vi "Write bool.vi"(0 "OWEN HMI in":refnum<class "OWEN HMI.lvclass">, 5 "Bool":T1, 11 "error in (no error)":errorcluster) -> (4 "OWEN HMI out":refnum<class "OWEN HMI.lvclass">, 15 "error out":errorcluster)   [LabVIEW 2019, in "OWEN HMI.lvclass"]
uses:
  OWEN HMI.lvclass
  Bool data.ctl
  OWEN HMI.lvclass/OWEN HMI.ctl
  <vilib>/NI/Modbus Library/API/Master/Modbus Master.lvclass
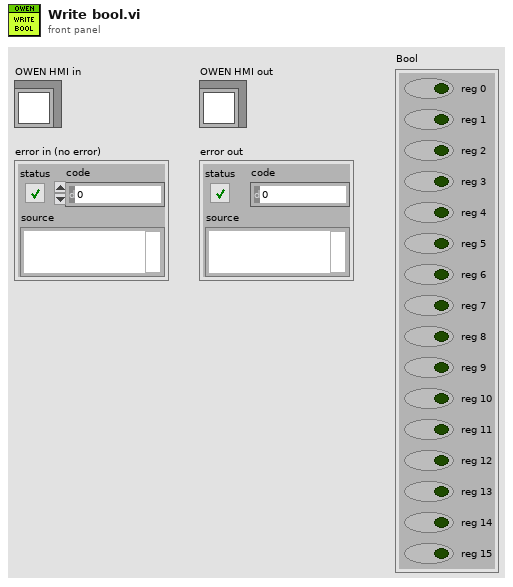
[diagram p1: front panel]
types:
  T1 = typedef "OWEN HMI.lvclass/Bool data.ctl" = cluster{"reg 0":bool, "reg 1":bool, "reg 2":bool, "reg 3":bool, "reg 4":bool, "reg 5":bool, "reg 6":bool, "reg 7":bool, "reg 8":bool, "reg 9":bool, "reg 10":bool, "reg 11":bool, "reg 12":bool, "reg 13":bool, "reg 14":bool, "reg 15":bool}
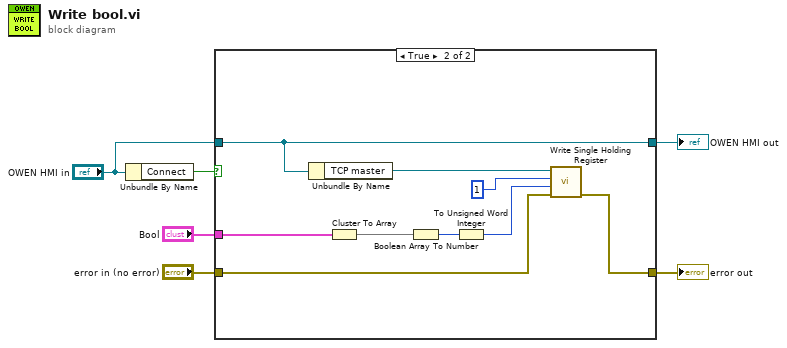
[diagram p0: block diagram]
diagram:
  n1 = Unbundle By Name("OWEN HMI in") -> ("Connect"=w6:bool)
  n2 = case shown="True" w6 {
    tunnel: "error in (no error)" -> [w8 w10]
    tunnel: "OWEN HMI in" -> [w7 w17]
    tunnel: [w7 w17] -> w3
    tunnel: [w8 w9] -> w2
    tunnel: "Bool" -> [_ w14]
    frame False {
    }
    frame True {
      n3 = Unbundle By Name(w17) -> ("TCP master"=w16:refnum<class "Modbus Master.lvclass">)
      n4 = Cluster To Array(cluster=w14) -> (array=w13:bool[])
      n5 = Boolean Array To Number(Boolean array=w13) -> (number=w12:u32)
      n6 = To Unsigned Word Integer(number=w12) -> (unsigned 16bit integer=w11:u16)
      n7 = call-dynamic "Write Single Holding Register.vi"("error in"=w10, "register to write"=w11, "address"=u16 1, "Modbus master in"=w16) -> ("error out"=w9:errorcluster)  [unwired: 6 in, 1 out]
    }
  }
  "OWEN HMI out" <- w3
  "error out" <- w2
